vi "Set Manual Range and Resolution.vi"(8 "error in (no error)":errorcluster, 9 "Resolution":dbl, 10 "Range":dbl, 11 "3446X in":refnum<class "3446X.lvclass">) -> (0 "error out":errorcluster, 3 "3446X out":refnum<class "3446X.lvclass">)   [LabVIEW 2018, in "3446X.lvlib" / "3446X.lvclass"]
uses:
  3446X.lvclass
  PPLs/DMM/Parent/DMM.lvlibp/DMM.lvclass
  C:/Projects/LabVIEW/PPLs/DMM/Parent/DMM.lvlibp/DMM.lvclass
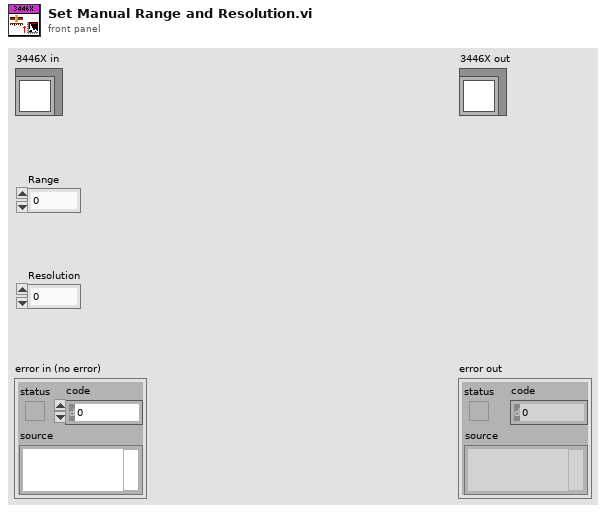
[diagram p1: front panel]
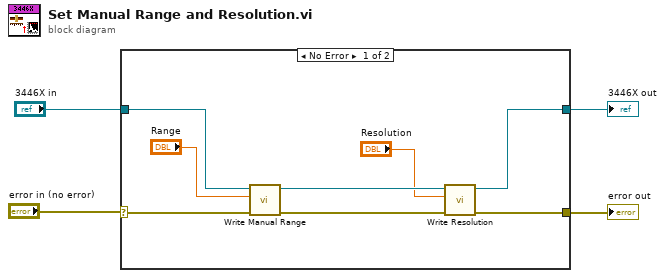
[diagram p0: block diagram]
diagram:
  n1 = case shown="No Error" "error in (no error)" {
    selector: "error in (no error)" -> [w12 w13]
    tunnel: "3446X in" -> [w11 w14]
    tunnel: [w6 w14] -> w2
    tunnel: [w5 w13] -> w1
    frame No Error {
      n2 = call "Write Manual Range.vi"("error in (no error)"=w12, "Manual Range"="Range", "DMM in"=w11) -> ("error out"=w8:errorcluster, "DMM out"=w9:refnum<class "3446X.lvclass">)  [unwired: 7 in]
      n3 = call "Write Resolution.vi"("error in (no error)"=w8, "Resolution"="Resolution", "DMM in"=w9) -> ("error out"=w5:errorcluster, "DMM out"=w6:refnum<class "3446X.lvclass">)  [unwired: 7 in]
    }
    frame Error {
    }
  }
  "error out" <- w1
  "3446X out" <- w2
